vi "libssh2_session_get_blocking.vi"(8 "error in (no error)":errorcluster, 11 "session":T1) -> (0 "error out":errorcluster, 2 "blocking":bool)   [LabVIEW 2013, in "libssh2.lvlib"]
doc: "Gets the blocking mode on the session."
uses:
  libssh2.lvlib
  Session Refnum.ctl
  Not A Session.vi
  <vilib>/Utility/error.llb/Error Cluster From Error Code.vi
  Global Settings.vi
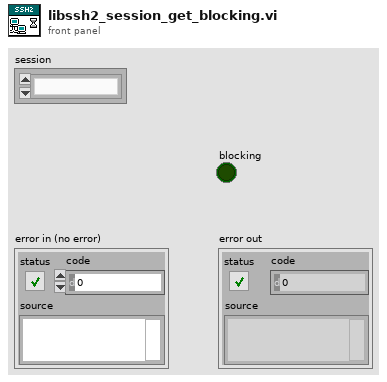
[diagram p1: front panel]
types:
  T1 = typedef "libssh2.lvlib/Session Refnum.ctl" = refnum<k1>
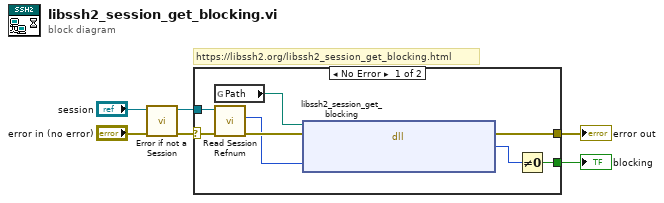
[diagram p0: block diagram]
diagram:
  # "https://libssh2.org/libssh2_session_get_blocking.html"
  n1 = call "Error if not a Session.vi"("error in (no error)"="error in (no error)", "session"="session") -> ("error out"=w3:errorcluster, "session out"=w1:T1)  [unwired: 8 in]
  n2 = case shown="No Error" w3 {
    selector: w3 -> [w13 w15]
    tunnel: [w14 w15] -> w6
    tunnel: w1 -> [w11 _]
    tunnel: [w12 _] -> w4
    frame No Error {
      n3 = global read "Global Settings.vi" "Path"() -> (w8:path)
      n4 = call "Read Session Refnum.vi"("error in (no error)"=w13, "session"=w11) -> ("error out"=w10:errorcluster, "LIBSSH2_SESSION*"=w9:u64)  [unwired: 8 in]
      n5 = dll-call lib="?" fn="libssh2_session_get_blocking"(path in=w8, error in=w10, "session"=w9) -> (error out=w14:errorcluster, "return value"=w7:i32)  [unwired: 2 in, 1 out]
      n6 = Not Equal To 0?(x=w7) -> (x != 0?=w12:bool)
    }
    frame Error {
    }
  }
  "error out" <- w6
  "blocking" <- w4
